vi "DHE_send_custom.vi"(7 "valid params":string[](array[string]), 8 "error in (no error)":errorcluster, 10 "args":string, 11 "fd":i32) -> (0 "error IO":errorcluster, 2 "str result":string, 3 "fd out":i32)   [LabVIEW 2016]
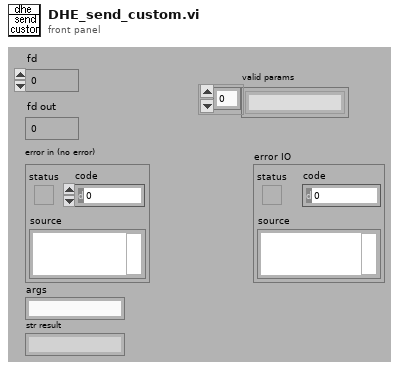
[diagram p1: front panel]
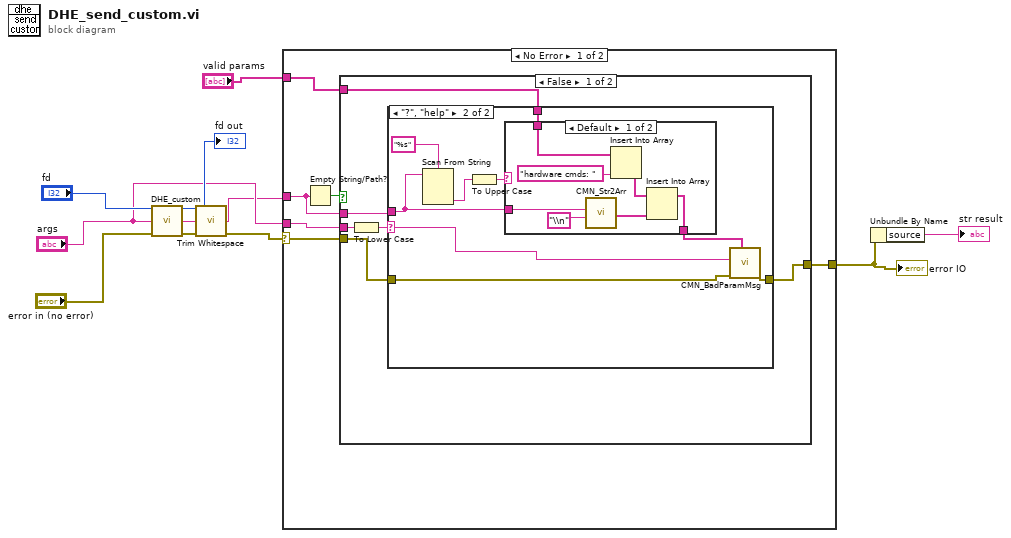
[diagram p0: block diagram]
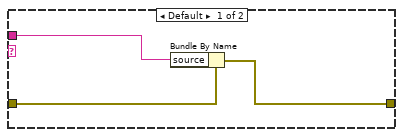
[diagram p2: hidden frame]
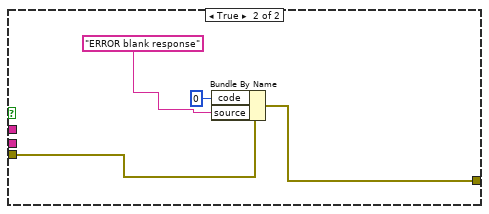
[diagram p4: hidden frame]
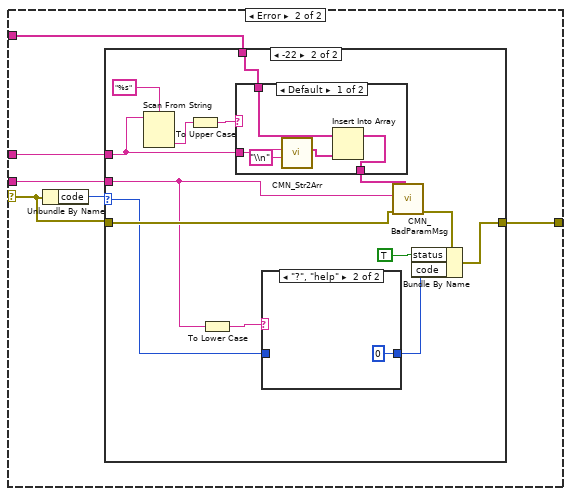
[diagram p5: hidden frame]
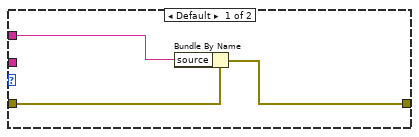
[diagram p6: hidden frame]
diagram:
  n1 = call "DHE_custom.vi"("fd"="fd", "args"="args", "error in (no error)"="error in (no error)") -> ("fd out"=→"fd out":i32, "str result"=w6:string, "error out"=w1:errorcluster)  [unwired: 10 out]
  n2 = call <vilib>:"Trim Whitespace.vi"("string"=w6) -> ("trimmed string"=w3:string)  [unwired: 1 in]
  n3 = case shown="No Error" w1 {
    selector: w1 -> [w16 w50]
    tunnel: "args" -> [w12 w52]
    tunnel: [w15 w49] -> w5
    tunnel: w3 -> [w13 w48]
    tunnel: "valid params" -> [w11 w47]
    frame No Error {
      n4 = Empty String/Path?(string/path=w13) -> (empty?=w14:bool)
      n5 = case shown="False" w14 {
        tunnel: w16 -> [w20 w46]
        tunnel: [w18 w45] -> w15
        tunnel: w13 -> [w19 _]
        tunnel: w12 -> [w22 _]
        tunnel: w11 -> [w17 _]
        frame False {
          n6 = To Lower Case(string=w22) -> (all lower case string=w21:string)
          n7 = case shown="\"?\", \"help\"" w21 {
            selector: w21 -> [_ w27]
            tunnel: w20 -> [w25 w29]
            tunnel: [w24 w26] -> w18
            tunnel: w19 -> [w23 w33]
            tunnel: w17 -> [_ w28]
            frame Default {
              n8 = Bundle By Name(cluster=w25, "source"=w23) -> (w24:errorcluster)
            }
            frame "?", "help" {
              n9 = Scan From String(format string="%s", input string=w33) -> (output 1=w31:string)  [unwired: 2 in, 4 out]
              n10 = To Upper Case(1:w31) -> (0:w30:string)
              n11 = case shown="Default" w30 {
                tunnel: [w39 w42] -> w34
                tunnel: w33 -> [w38 _]
                tunnel: w28 -> [w37 w42]
                frame Default {
                  n12 = call "CMN_Str2Arr.vi"("separator"="\\n", "string in"=w38) -> ("Array out"=w40:string[])  [unwired: 2 in, 7 out]
                  n13 = Insert Into Array(array=w37, new element="hardware cmds: " ("new element/subarray")) -> (w35:string[])  [unwired: 1 in]
                  n14 = Insert Into Array(array=w35, new element=w40) -> (w39:string[])  [unwired: 1 in]
                }
                frame "ERR", "ERROR" {
                }
              }
              n15 = call "CMN_BadParamMsg.vi"("valid params"=w34, "error in (no error)"=w29, "parameter"=w27) -> ("error out"=w26:errorcluster)  [unwired: 1 in, 7 out]
            }
          }
        }
        frame True {
          n16 = Bundle By Name(cluster=w46, "code"=0, "source"="ERROR blank response") -> (w45:errorcluster)
        }
      }
    }
    frame Error {
      n17 = Unbundle By Name(w50) -> ("code"=w51:i32)
      n18 = case shown="-22" w51 {
        selector: w51 -> [_ w59]
        tunnel: w52 -> [_ w60]
        tunnel: w50 -> [w55 w63]
        tunnel: [w54 w61] -> w49
        tunnel: w47 -> [_ w65]
        tunnel: w48 -> [w53 w68]
        frame Default {
          n19 = Bundle By Name(cluster=w55, "source"=w53) -> (w54:errorcluster)
        }
        frame -22 {
          n20 = Scan From String(format string="%s", input string=w68) -> (output 1=w66:string)  [unwired: 2 in, 4 out]
          n21 = To Upper Case(1:w66) -> (0:w64:string)
          n22 = To Lower Case(string=w60) -> (all lower case string=w57:string)
          n23 = case shown="Default" w64 {
            tunnel: [w74 w77] -> w69
            tunnel: w68 -> [w73 _]
            tunnel: w65 -> [w72 w77]
            frame Default {
              n24 = call "CMN_Str2Arr.vi"("separator"="\\n", "string in"=w73) -> ("Array out"=w75:string[])  [unwired: 2 in, 7 out]
              n25 = Insert Into Array(array=w72, new element=w75) -> (w74:string[])  [unwired: 1 in]
            }
            frame "ERR", "ERROR" {
            }
          }
          n26 = case shown="\"?\", \"help\"" w57 {
            tunnel: w59 -> [w70 _]
            tunnel: [w70 0 ("code")] -> w58
            frame Default {
            }
            frame "?", "help" {
            }
          }
          n27 = call "CMN_BadParamMsg.vi"("valid params"=w69, "error in (no error)"=w63, "parameter"=w60) -> ("error out"=w62:errorcluster)  [unwired: 1 in, 7 out]
          n28 = Bundle By Name(cluster=w62, "status"=TRUE, "code"=w58) -> (w61:errorcluster)
        }
      }
    }
  }
  "error IO" <- w5
  n29 = Unbundle By Name(w5) -> ("source"=→"str result":string)
